vi "UtilityLib.set color of boolean.vi"(0 "button":refnum<vi>, 2 "valueStatus":T1, 3 "nOfPair (0)":i32, 4 "setTRUEColor (FALSE)":bool, 5 "error in (no error)":errorcluster) -> (19 "error out":errorcluster)   [LabVIEW 2014, in "UtilityLib.lvlib"]
doc: "Changes the color of a boolean element to values defined in six-color vi.\n\nColor pairs include False, True, True to False, and False to True."
uses:
  UtilityLib.lvlib
  UtilityLib.valueStatus.ctl
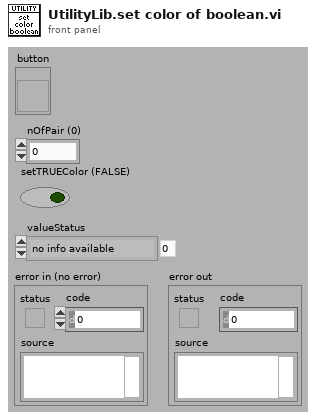
[diagram p1: front panel]
types:
  T1 = typedef "UtilityLib.lvlib/UtilityLib.valueStatus.ctl" = enum16{"no info available", "stand by/off", "on", "warning", "alarm/malfunction", "not implemented", "user action required", "important information", "system default", "control default", "indicator default", "button default"}
  T2 = cluster{"elementBackground":u32, "elementBackground":u32}
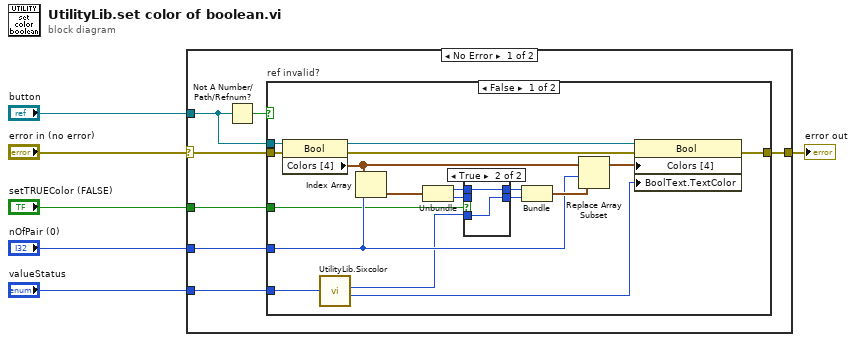
[diagram p0: block diagram]
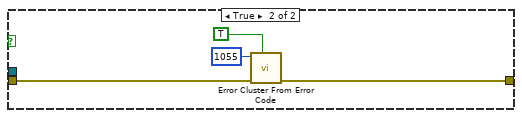
[diagram p3: hidden frame]
diagram:
  n1 = case shown="No Error" "error in (no error)" {
    selector: "error in (no error)" -> [w7 w40]
    tunnel: [w13 w40] -> w6
    tunnel: "valueStatus" -> [w11 _]
    tunnel: "nOfPair (0)" -> [w10 _]
    tunnel: "setTRUEColor (FALSE)" -> [w9 _]
    tunnel: "button" -> [w8 _]
    frame No Error {
      n2 = Not A Number/Path/Refnum?(number/path/refnum=w8) -> (NaN/Path/Refnum?=w12:bool)
      n3 = case "ref invalid?" shown="False" w12 {
        tunnel: [w30 w38] -> w13
        tunnel: w7 -> [w28 w39]
        tunnel: w8 -> [w29 _]
        tunnel: w11 -> [w31 _]
        tunnel: w10 -> [w20 _]
        tunnel: w9 -> [w19 _]
        frame False {
          n4 = property class="Bool"(reference=w29, error in=w28) -> (reference out=w27:refnum<vi>, error out=w26:errorcluster, "Colors [4]"=w24:cluster{u32, u32}[])
          n5 = call "UtilityLib.Sixcolor.vi"("State"=w31) -> ("elementBackground"=w18:u32, "elementText"=w21:u32)  [unwired: 2 in, 2 out]
          n6 = Index Array(array=w24, index=w20) -> (element=w25:cluster{u32, u32})
          n7 = Unbundle(w25) -> (w16:u32, w14:u32)
          n8 = case shown="True" w19 {
            tunnel: w18 -> [w33 w35]
            tunnel: [w32 w35] -> w17
            tunnel: [w33 w34] -> w15
            tunnel: w16 -> [_ w34]
            tunnel: w14 -> [w32 _]
            frame False {
            }
            frame True {
            }
          }
          n9 = Bundle("elementBackground"=w15, "elementBackground"=w17) -> (w23:T2)  [unwired: 1 in]
          n10 = Replace Array Subset(array=w24, new element=w23, index=w20) -> (w22:cluster{u32, u32}[])
          n11 = property class="Bool"(reference=w27, error in=w26, "Colors [4]"=w22, "BoolText.TextColor"=w21) -> (error out=w30:errorcluster)  [unwired: 1 out]
        }
        frame True {
          n12 = call <vilib>:"Error Cluster From Error Code.vi"("show call chain? (False)"=TRUE, "error in (no error)"=w39, "error code (0)"=1055) -> ("error out"=w38:errorcluster)  [unwired: 6 in]
        }
      }
    }
    frame Error {
    }
  }
  "error out" <- w6
